vi "decode_statis_id.vi"(11 "satatus_id":u32) -> (0 "Alarm":bool, 1 "Error":bool, 2 "Standby":bool, 3 "Operational":bool)   [LabVIEW 2014]
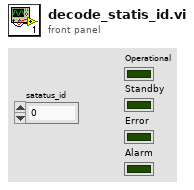
[diagram p1: front panel]
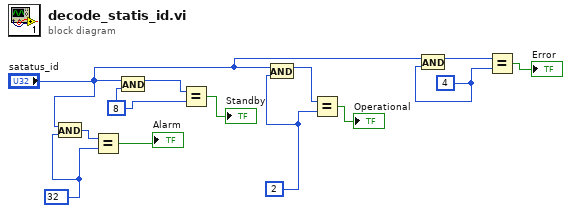
[diagram p0: block diagram]
diagram:
  w13 = u32 4 ("y")
  w10 = u32 2 ("y")
  w6 = u32 8 ("y")
  w8 = u32 32 ("y")
  n1 = And(x="satatus_id", y=w8) -> (x .and. y?=w7:u32)
  n2 = Equal?(x=w7, y=w8) -> (x = y?=→"Alarm":bool)
  n3 = And(x="satatus_id", y=w6) -> (x .and. y?=w5:u32)
  n4 = Equal?(x=w5, y=w6) -> (x = y?=→"Standby":bool)
  n5 = And(x="satatus_id", y=w10) -> (x .and. y?=w9:u32)
  n6 = Equal?(x=w9, y=w10) -> (x = y?=→"Operational":bool)
  n7 = And(x="satatus_id", y=w13) -> (x .and. y?=w12:u32)
  n8 = Equal?(x=w12, y=w13) -> (x = y?=→"Error":bool)
